vi "Close.vi"(2 "error in":errorcluster, 3 "VISA arduino in":refnum<visa-resource-name>) -> (0 "error out":errorcluster)   [LabVIEW 2021]
uses:
  Delay_Global.vi
  <vilib>/Utility/error.llb/Error Cluster From Error Code.vi
  <vilib>/ErrorRing/Error Ring.xnode
panel:
  out "ext delay":u32
  # "Private"
  # "Public"
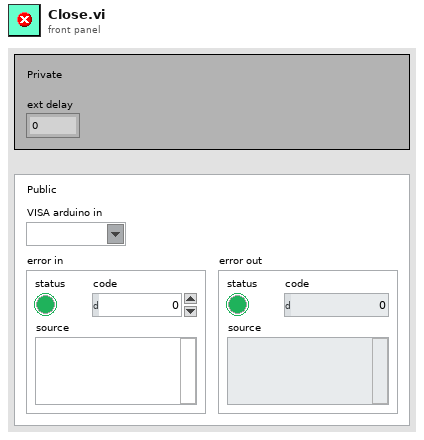
[diagram p1: front panel]
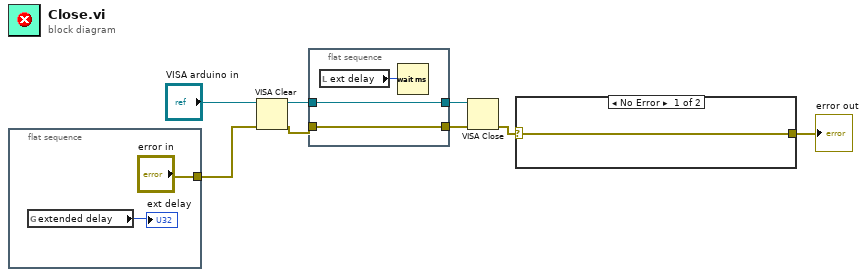
[diagram p0: block diagram]
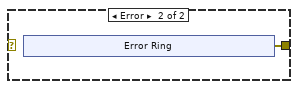
[diagram p2: hidden frame]
diagram:
  n1 = flat-sequence {
    tunnel: ["error in"] -> w1
    frame #0 {
      n2 = global read "Delay_Global.vi" "extended delay"() -> (→"ext delay":u32)
    }
  }
  n3 = VISA Clear(VISA resource name="VISA arduino in", error in (no error)=w1) -> (VISA resource name out=w7:refnum<visa-resource-name>, error out=w8:errorcluster)
  n4 = flat-sequence {
    tunnel: [w13] -> w5
    tunnel: w7 -> [w13]
    tunnel: [w12] -> w6
    tunnel: w8 -> [w12]
    frame #0 {
      n5 = local read "ext delay"() -> (w11:u32)
      n6 = Wait (ms)(milliseconds to wait=w11) -> ()  [unwired: 1 out]
    }
  }
  n7 = VISA Close(VISA resource name=w5, error in (no error)=w6) -> (error out=w4:errorcluster)
  n8 = case shown="No Error" w4 {
    selector: w4 -> [w14 _]
    tunnel: [w14 w15] -> w3
    frame No Error {
    }
    frame Error {
      n9 = xnode "Error Ring"() -> ("error out"=w15:errorcluster)
    }
  }
  "error out" <- w3
